vi "Color Tracking Table.vi"(5 "Mode":enum16{"Select", "Track"}(ring), 9 "TrackingTableColors":i32[][](array[numeric]), 10 "TrackingRowsSelected":i32[](array[numeric]), 11 "Tracking Table Ref":refnum<vi>) -> ()   [LabVIEW 2013]
uses:
  <vilib>/Utility/miscctls.llb/LVRowAndColumnTypeDef.ctl
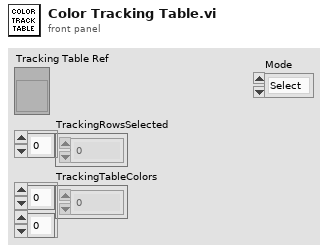
[diagram p1: front panel]
types:
  T1 = typedef "LVRowAndColumnTypeDef.ctl" = cluster{"Row":i32, "Column":i32}
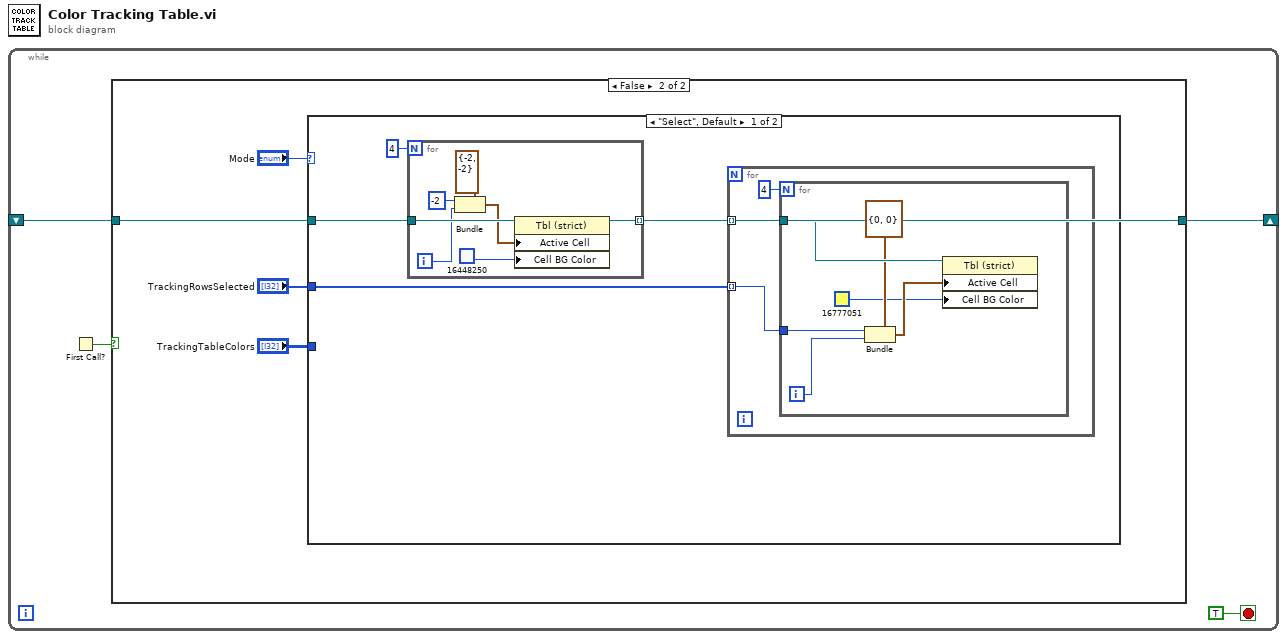
[diagram p0: block diagram]
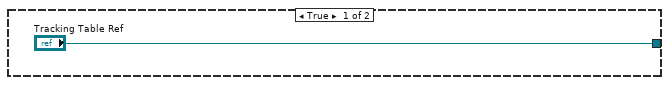
[diagram p2: hidden frame]
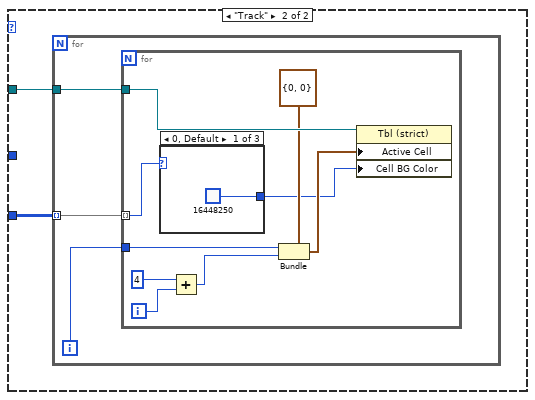
[diagram p3: hidden frame]
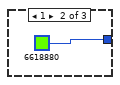
[diagram p4: hidden frame]
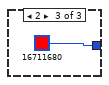
[diagram p5: hidden frame]
diagram:
  n1 = while {
    shift-right: [w3] -> _
    shift-left: _ -> [w2]
    stop <- TRUE stop-if-true
    n2 = First Call?() -> (First Call?: T/F=w4:bool)
    n3 = case shown="False" w4 {
      tunnel: w2 -> [_ w6]
      tunnel: ["Tracking Table Ref" w6] -> w3
      frame True {
      }
      frame False {
        n4 = case shown="\"Select\", Default" "Mode" {
          tunnel: "TrackingTableColors" -> [_ w31]
          tunnel: w6 -> [w12 w30]
          tunnel: "TrackingRowsSelected" -> [w13 _]
          frame "Select", Default {
            n5 = for {
              N: 4 -> [_]
              tunnel: w12 -> [w20]
              tunnel: [w19] -> w11 mode=indexing
              i -> [w14]
              n6 = Bundle(cluster=T1 {"Row"=-2, "Column"=-2} ("Active Cell:Active Cell"), "Row"=-2, "Column"=w14) -> (w15:T1)
              n7 = property class="Tbl (strict)"(reference=w20, "Active Cell"=w15, "Cell BG Color"=u32 16448250) -> (reference out=w19:refnum<vi>)  [unwired: 1 in, 1 out]
            }
            n8 = for {
              tunnel: w13 -> [w21] mode=indexing
              tunnel: w11 -> [w23] mode=indexing
              n9 = for {
                N: 4 -> [_]
                tunnel: w23 -> [w29]
                tunnel: w21 -> [w27]
                i -> [w25]
                n10 = Bundle(cluster=T1 {"Row"=0, "Column"=0} ("Active Cell:Active Cell"), "Row"=w27, "Column"=w25) -> (w26:T1)
                n11 = property class="Tbl (strict)"(reference=w29, "Active Cell"=w26, "Cell BG Color"=u32 16777051) -> ()  [unwired: 1 in, 2 out]
              }
            }
          }
          frame "Track" {
            n12 = for {
              tunnel: w31 -> [w34] mode=indexing
              tunnel: w30 -> [w33]
              i -> [w32]
              n13 = for {
                tunnel: w34 -> [w36] mode=indexing
                tunnel: w33 -> [w43]
                tunnel: w32 -> [w41]
                i -> [w39]
                n14 = case shown="0, Default" w36 {
                  tunnel: [u32 16448250 u32 6618880 u32 16711680] -> w35
                  frame 0, Default {
                  }
                  frame 1 {
                  }
                  frame 2 {
                  }
                }
                n15 = Add(x=4, y=w39) -> (x+y=w40:i32)
                n16 = Bundle(cluster=T1 {"Row"=0, "Column"=0} ("Active Cell:Active Cell"), "Row"=w41, "Column"=w40) -> (w37:T1)
                n17 = property class="Tbl (strict)"(reference=w43, "Active Cell"=w37, "Cell BG Color"=w35) -> ()  [unwired: 1 in, 2 out]
              }
            }
          }
        }
      }
    }
  }
